vi "Get Aligned Image Transfer Size.vi"(9 "Y Resolution":u32, 10 "X Resolution":u32, 11 "Image Transfer Size Alignment":u32=1 min=1) -> (3 "Aligned Image Transfer Size":u64)   [LabVIEW 2017, in "NI_VDM_FPGA_Basics.lvlib"]
uses:
  <vilib>/visionFPGA/NI_VDM_FPGA_Basics.lvlib
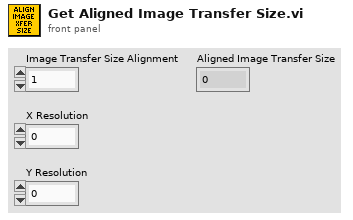
[diagram p1: front panel]
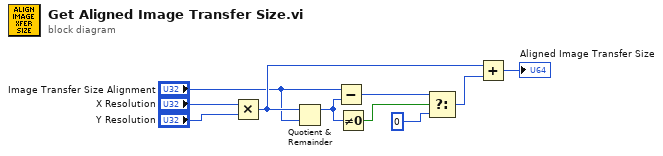
[diagram p0: block diagram]
diagram:
  n1 = Multiply(x="X Resolution", y="Y Resolution") -> (x*y=w8:u32)
  n2 = Quotient & Remainder(x=w8, y="Image Transfer Size Alignment") -> (x-y*floor(x/y)=w6:u32)  [unwired: 1 out]
  n3 = Subtract(x="Image Transfer Size Alignment", y=w6) -> (x-y=w5:u32)
  n4 = Not Equal To 0?(x=w6) -> (x != 0?=w3:bool)
  n5 = Select(t=w5, s=w3, f=u32 0) -> (s? t:f=w9:u32)
  n6 = Add(x=w8, y=w9) -> (x+y=→"Aligned Image Transfer Size":u32)
